vi "VSI Write Read Bits.vi"(6 "ReadBitsNum":i32, 7 "pWriteBitStr":string, 8 "error in (no error)":errorcluster, 9 "SPIIndex":i32, 10 "DevIndex":i32, 11 "DevType":i32) -> (0 "error out":errorcluster, 2 "function return":i32, 3 "pReadBitStr":string)   [LabVIEW 2012, in "ControlSPI.lvlib"]
doc: "int WINAPI VSI_WriteReadBits(int DevType,int DevIndex,int SPIIndex,unsigned char *pWriteBitStr,unsigned char *pReadBitStr,int ReadBitsNum);"
uses:
  ControlSPI.lvlib
  Ginkgo_Driver.dll
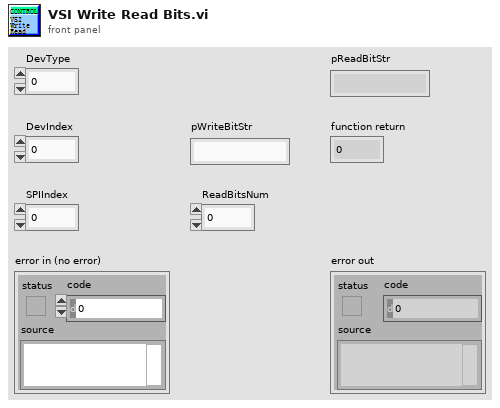
[diagram p1: front panel]
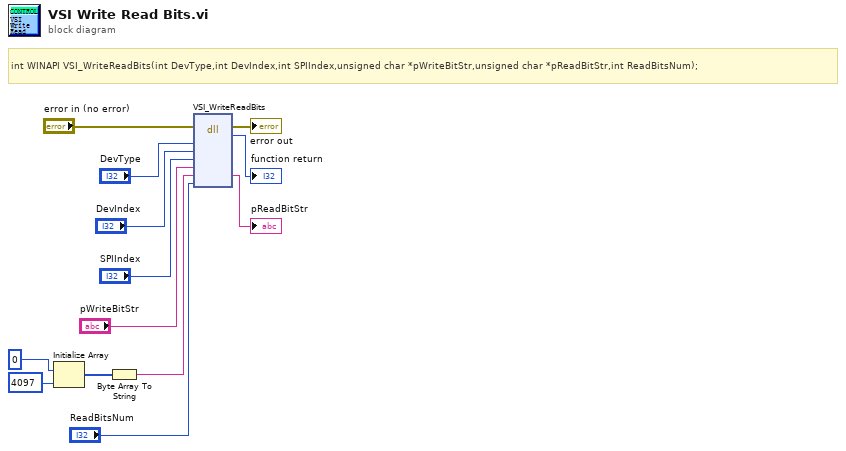
[diagram p0: block diagram]
diagram:
  # "int WINAPI VSI_WriteReadBits(int DevType,int DevIndex,int SPIIndex,unsigned char *pWriteBitStr,unsigned char *pReadBitStr,int ReadBitsNum);"
  n1 = Initialize Array(u8 0 ("element"), 4097 ("dimension size")) -> (w8:u8[])
  n2 = Byte Array To String(unsigned byte array=w8) -> (string=w7:string)
  n3 = dll-call lib="E:/Project/vt_ginkgo/truck/Ginkgo Driver/vs2010/Ginkgo_USB-I2C_API_v2.0.3.0/lib/labview_32bit/ControlSPI/Ginkgo_Driver.*" fn="VSI_WriteReadBits"(error in="error in (no error)", "DevType"="DevType", "DevIndex"="DevIndex", "SPIIndex"="SPIIndex", "pWriteBitStr"="pWriteBitStr", "pReadBitStr"=w7, "ReadBitsNum"="ReadBitsNum") -> (error out=→"error out":errorcluster, →"function return":i32, "pReadBitStr"=→"pReadBitStr":string)  [unwired: 7 in, 1 out]
